vi "UI trackingXY CUDA_perROI.vi"() -> ()   [LabVIEW 2017]
uses:
  <vilib>/vision/Image Controls.llb/IMAQ Image.ctl
  control/Bead track.ctl
panel:
  in  "beads track":T1[](array[typedef]) {"centroid"."Y Centroid" format="%.2f"; "centroid"."X Centroid" format="%.2f"; "ROI Des out"."Contours"."Type" items=["No Selection", "Point", "Line", "Rectangle", "Oval", "Polygon", "Freehand Region", "Annulus", "Unused2", "Unused3", "Broken Line", "Freehand Line", "Rotated Rectangle"]}
  out "rdp_mean":dbl[][](array[numeric])
  out "tracking out":T1[](array[typedef]) {"centroid"."Y Centroid" format="%.2f"; "centroid"."X Centroid" format="%.2f"; "ROI Des out"."Contours"."Type" items=["No Selection", "Point", "Line", "Rectangle", "Oval", "Polygon", "Freehand Region", "Annulus", "Unused2", "Unused3", "Broken Line", "Freehand Line", "Rotated Rectangle"]}
  in  "Centroid":cluster{"X Centroid":sgl, "Y Centroid":sgl} {"Y Centroid" format="%.2f"; "X Centroid" format="%.2f"}
  out "x_qi_out":sgl[][](array[numeric])
  out "y_qi_out":sgl[][](array[numeric])
  out "rdp_profile":sgl[][][](array[numeric])
  in  "image ref":T3[](array[typedef])
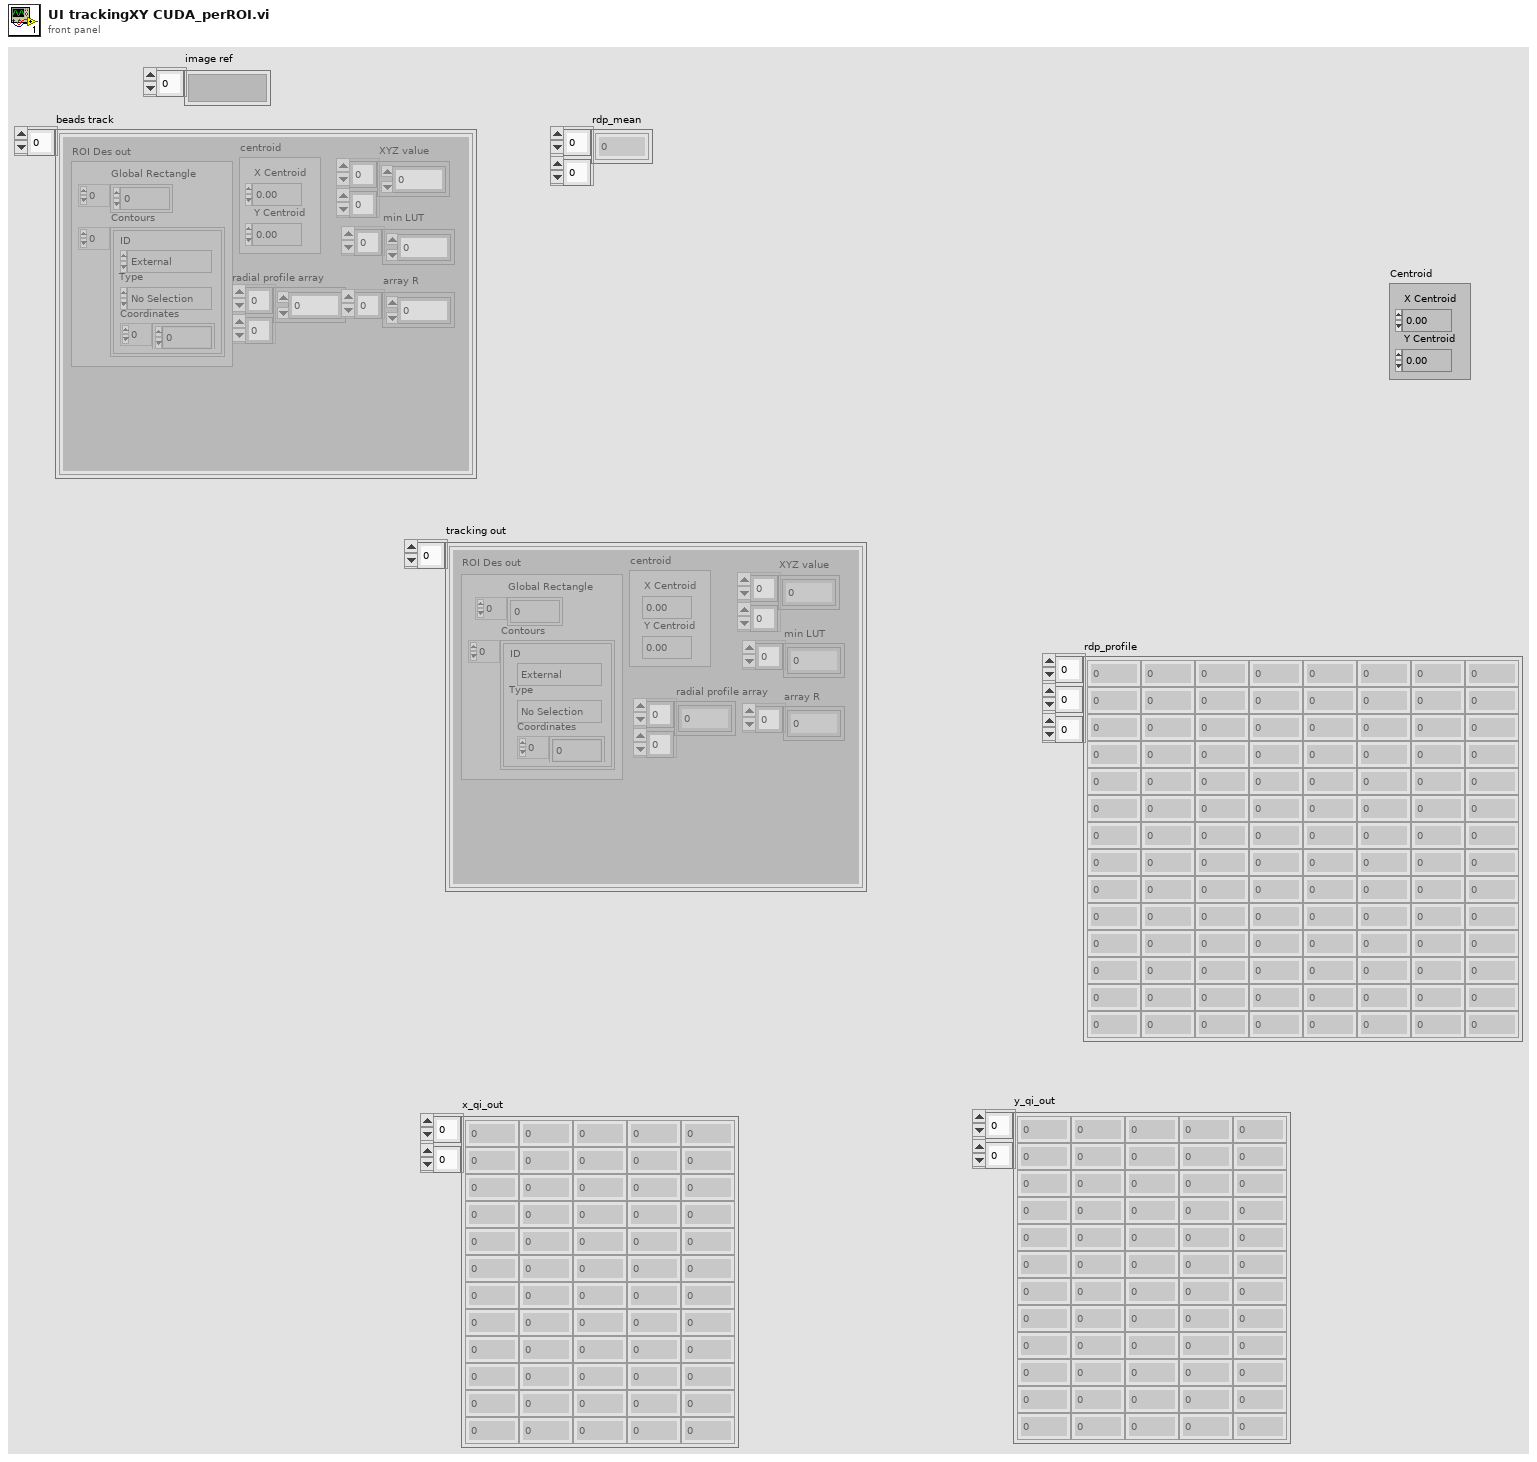
[diagram p1: front panel]
types:
  T1 = typedef "Bead track.ctl" = cluster{"XYZ value":dbl[][], "radial profile array":dbl[][], "min LUT":dbl[], "ROI Des out":T2, "array R":dbl[], "centroid":cluster{"X Centroid":sgl, "Y Centroid":sgl}}
  T2 = typedef "ROI Descriptor" = cluster{"Global Rectangle":i32[], "Contours":cluster{"ID":enum32{"External", "Internal"}, "Type":u32, "Coordinates":i32[]}[]}
  T3 = typedef "IMAQ Image.ctl" = refnum<image>
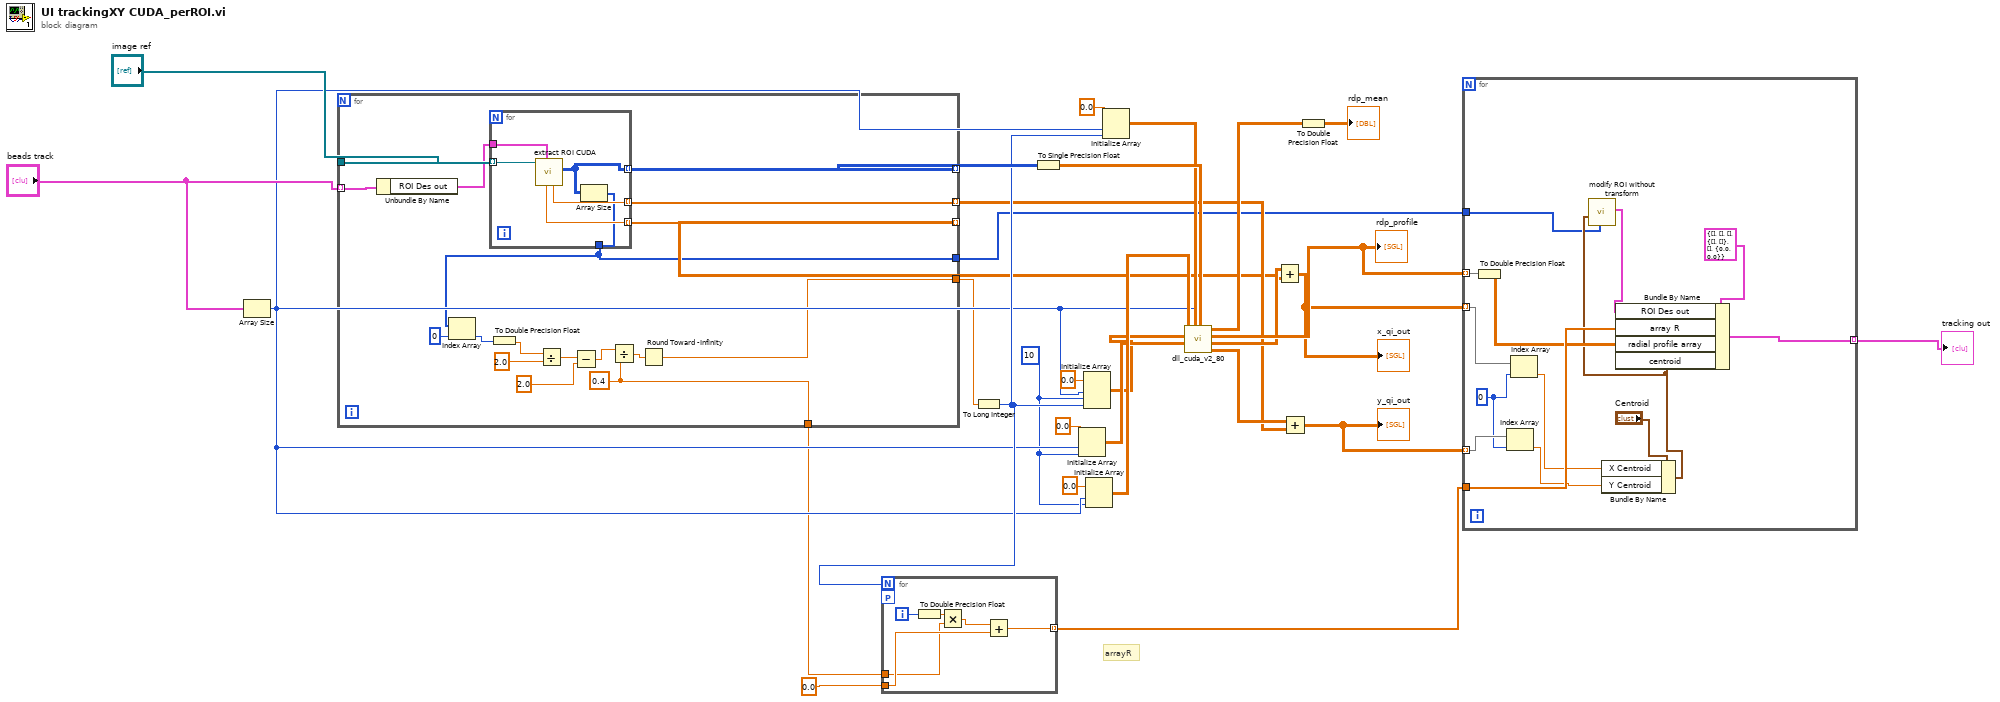
[diagram p0: block diagram]
diagram:
  w4 = 10 ("n_frame")
  # "arrayR"
  n1 = Array Size(array="beads track") -> (size(s)=w5:i32)
  n2 = for {
    tunnel: "image ref" -> [w47]
    tunnel: [w46] -> w26 mode=indexing
    tunnel: [w45] -> w7 mode=indexing
    tunnel: [w44] -> w8 mode=indexing
    tunnel: "beads track" -> [w43] mode=indexing
    tunnel: [w33] -> w3
    tunnel: [w32] -> w2
    tunnel: [w31] -> w1
    w32 = 0.4 ("y")
    n3 = Unbundle By Name(w43) -> ("ROI Des out"=w42:T2)
    n4 = for {
      tunnel: w47 -> [w53] mode=indexing
      tunnel: [w48] -> w46 mode=indexing
      tunnel: [w52] -> w45 mode=indexing
      tunnel: [w51] -> w44 mode=indexing
      tunnel: [w50] -> w31
      tunnel: w42 -> [w49]
      n5 = call "extract ROI CUDA.vi"("ROI Descriptor"=w49, "CCD image ref"=w53) -> ("ROI array out"=w48:u8[][], "Y_base"=w51:sgl, "X_base"=w52:sgl)  [unwired: 7 in]
      n6 = Array Size(array=w48) -> (size(s)=w50:i32[])
    }
    n7 = Index Array(array=w31, index=0) -> (element=w41:i32)
    n8 = To Double Precision Float(number=w41) -> (double precision float=w37:dbl)
    n9 = Divide(x=w37, y=2.0) -> (x/y=w38:dbl)
    n10 = Subtract(x=w38, y=2.0) -> (x-y=w39:dbl)
    n11 = Divide(x=w39, y=w32) -> (x/y=w40:dbl)
    n12 = Round Toward -Infinity(1:w40) -> (0:w33:dbl)
  }
  n13 = To Long Integer(number=w3) -> (32bit integer=w13:i32)
  n14 = for "For循环" {
    N: w13 -> [_]
    tunnel: 0.0 ("R_min") -> [w57]
    tunnel: [w55] -> w17 mode=indexing
    workers-P: _ -> [_]
    tunnel: w2 -> [w54]
    i -> [w59]
    n15 = To Double Precision Float(number=w59) -> (double precision float=w56:dbl)
    n16 = Multiply(x=w56, y=w54) -> (x*y=w58:dbl)
    n17 = Add(x=w58, y=w57) -> (x+y=w55:dbl)
  }
  n18 = To Single Precision Float(number=w26) -> (single precision float=w25:sgl[][][][])
  n19 = Initialize Array(sgl 0.0 ("element"), w5, w4) -> (w24:sgl[][])
  n20 = Initialize Array(sgl 0.0 ("element"), w5, w4, w13) -> (w23:sgl[][][])
  n21 = Initialize Array(sgl 0.0 ("element"), w5, w4) -> (w27:sgl[][])
  n22 = Initialize Array(sgl 0.0 ("element"), w5, w13) -> (w12:sgl[][])
  n23 = call "dll_cuda_v2_80.vi"("n_stream"=w5, "rdp_mean"=w12, "yc"=w27, "xc"=w24, "rdp_profile"=w23, "img_mat 4d"=w25) -> ("yc out"=w22:sgl[][], "xc out"=w16:sgl[][], "rdp_profile out"=w20:sgl[][][], "rdp_mean out"=w10:sgl[][])  [unwired: 2 in]
  "rdp_profile" <- w20
  n24 = Add(x=w16, y=w7) -> (x+y=w19:sgl[][])
  "x_qi_out" <- w19
  n25 = Add(x=w22, y=w8) -> (x+y=w18:sgl[][])
  "y_qi_out" <- w18
  n26 = To Double Precision Float(number=w10) -> (double precision float=→"rdp_mean":dbl[][])
  n27 = for {
    tunnel: w20 -> [w71] mode=indexing
    tunnel: w19 -> [w69] mode=indexing
    tunnel: w18 -> [w68] mode=indexing
    tunnel: w17 -> [w72]
    tunnel: w1 -> [w62]
    tunnel: [w60] -> w11 mode=indexing
    w67 = 0
    n28 = To Double Precision Float(number=w71) -> (double precision float=w70:dbl[][])
    n29 = Index Array(array=w68, index=w67) -> (element=w64:sgl)
    n30 = Index Array(array=w69, index=w67) -> (element=w65:sgl)
    n31 = Bundle By Name(cluster="Centroid", "X Centroid"=w65, "Y Centroid"=w64) -> (w63:cluster{"X Centroid":sgl, "Y Centroid":sgl})
    n32 = call "modify ROI without transform.vi"("ROI size num"=w62, "new x y"=w63) -> ("ROI Descriptor out"=w61:T2)  [unwired: 8 in, 1 out]
    n33 = Bundle By Name(cluster=T1 {"XYZ value"=[], "radial profile array"=[], "min LUT"=[], "ROI Des out"={"Global Rectangle"=[], "Contours"=[]}, "array R"=[], "centroid"={"X Centroid"=0.0, "Y Centroid"=0.0}} ("tracking"), "ROI Des out"=w61, "array R"=w72, "radial profile array"=w70, "centroid"=w63) -> (w60:T1)
  }
  "tracking out" <- w11
